vi "SetupCreateObjectFromTree.vi"(8 "error in":errorcluster, 11 "TreeControl in":refnum<vi>) -> (0 "error out":errorcluster, 3 "Setup out":refnum<class "Setup.lvclass">)   [LabVIEW 2013, in "DataCreation.lvlib"]
uses:
  DataCreation.lvlib
  classes/Datastructure/Setup/Setup.lvclass
  classes/Datastructure/Image/img.lvclass
  classes/Datastructure/Device/Device.lvclass
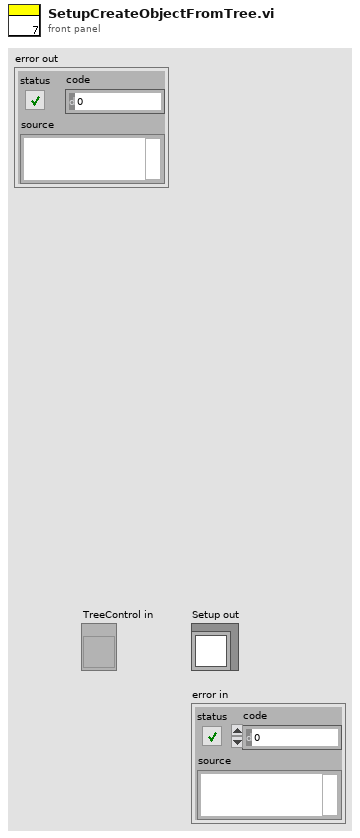
[diagram p1: front panel]
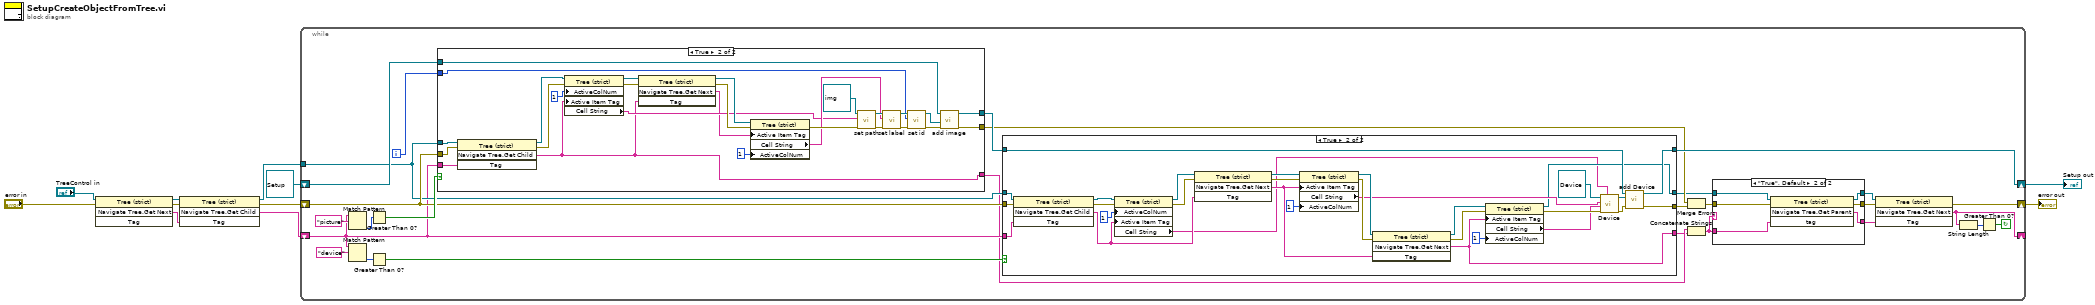
[diagram p0: block diagram]
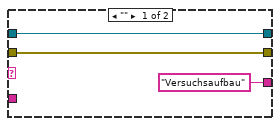
[diagram p2: hidden frame]
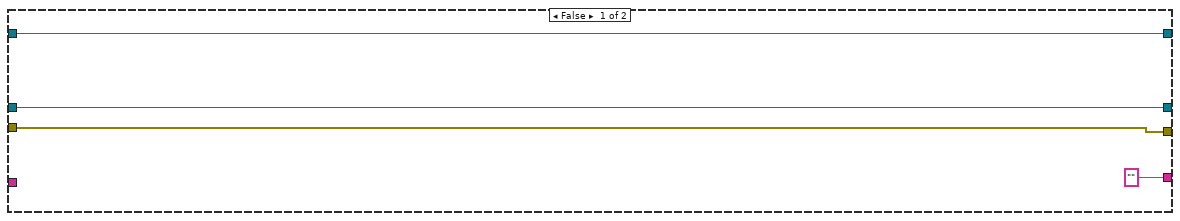
[diagram p3: hidden frame]
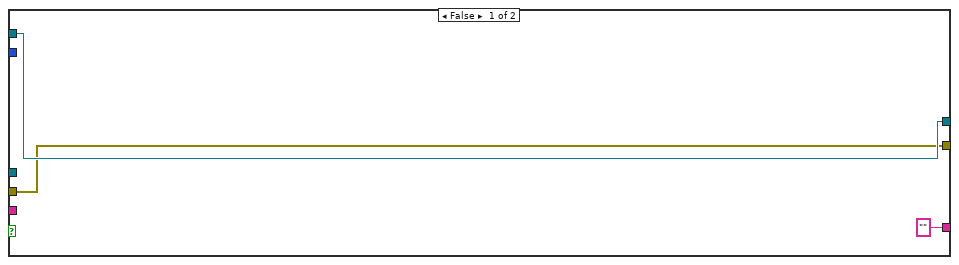
[diagram p4: hidden frame]
diagram:
  n1 = invoke class="Tree (strict)" method="Navigate Tree.Get Next"(reference="TreeControl in", error in="error in") -> (reference out=w6:refnum<vi>, error out=w7:errorcluster, "Navigate Tree:Get Next Item"=w8:string)  [unwired: 2 in, 1 out]
  n2 = invoke class="Tree (strict)" method="Navigate Tree.Get Child"(reference=w6, error in=w7, "Tag"=w8) -> (reference out=w11:refnum<vi>, error out=w9:errorcluster, "Navigate Tree:Get Child"=w10:string)  [unwired: 1 in, 1 out]
  n3 = while {
    shift-right: [w16] -> w1
    shift-left: w9 -> [w32]
    shift-right: [w25] -> w3
    shift-left: refnum<class "Setup.lvclass"> refnum ("Setup Ausgang") -> [w31]
    shift-right: [w14] -> _
    shift-left: w10 -> [w29]
    tunnel: w11 -> [w30]
    i -> [w12]
    stop <- w19 continue-if-true
    n4 = Match Pattern(string=w29, regular expression="picture" ("Regulärer Ausdruck")) -> (offset past match=w37:i32)  [unwired: 1 in, 3 out]
    n5 = Match Pattern(string=w29, regular expression="device" ("Regulärer Ausdruck")) -> (offset past match=w33:i32)  [unwired: 1 in, 3 out]
    n6 = Greater Than 0?(x=w37) -> (x > 0?=w36:bool)
    n7 = Greater Than 0?(x=w33) -> (x > 0?=w35:bool)
    n8 = case shown="True" w36 {
      tunnel: w29 -> [_ w92]
      tunnel: w32 -> [w82 w93]
      tunnel: w30 -> [_ w94]
      tunnel: [w82 w98] -> w24
      tunnel: w31 -> [w83 w97]
      tunnel: [w83 w91] -> w26
      tunnel: ["" ("Navigate Tree:Get Child") w90] -> w28
      tunnel: w12 -> [_ w87]
      frame False {
      }
      frame True {
        n9 = invoke class="Tree (strict)" method="Navigate Tree.Get Child"(reference=w94, error in=w93, "Tag"=w92) -> (reference out=w96:refnum<vi>, error out=w95:errorcluster, "Navigate Tree:Get Child"=w90:string)  [unwired: 1 in, 1 out]
        n10 = property class="Tree (strict)"(reference=w96, error in=w95, "ActiveColNum"=1 ("Active Cell:Active Column Number"), "Active Item Tag"=w90) -> (reference out=w106:refnum<vi>, error out=w107:errorcluster, "Cell String"=w102:string)
        n11 = invoke class="Tree (strict)" method="Navigate Tree.Get Next"(reference=w106, error in=w107, "Tag"=w90) -> (reference out=w105:refnum<vi>, error out=w104:errorcluster, "Navigate Tree:Get Next Item"=w101:string)  [unwired: 1 in, 1 out]
        n12 = property class="Tree (strict)"(reference=w105, error in=w104, "Active Item Tag"=w101, "ActiveColNum"=1 ("Active Cell:Active Column Number")) -> (error out=w111:errorcluster, "Cell String"=w103:string)  [unwired: 1 out]
        n13 = call-dynamic "set path.vi"("error in (no error)"=w111, "path"=w102, "img (Eingang)"=refnum<class "img.lvclass"> refnum ("img.lvclass")) -> ("error out"=w110:errorcluster, "img (Ausgang)"=w108:refnum<class "img.lvclass">)  [unwired: 7 in]
        n14 = call-dynamic "set label.vi"("error in (no error)"=w110, "label"=w103, "img (Eingang)"=w108) -> ("error out"=w88:errorcluster, "img (Ausgang)"=w89:refnum<class "img.lvclass">)  [unwired: 7 in]
        n15 = call-dynamic "set id.vi"("error in (no error)"=w88, "id"=w87, "img in"=w89) -> ("error out"=w86:errorcluster, "img out"=w85:refnum<class "img.lvclass">)  [unwired: 7 in]
        n16 = call-dynamic "add image.vi"("error in (no error)"=w86, "img.lvclass"=w85, "Setup (Eingang)"=w97) -> ("error out"=w98:errorcluster, "Setup (Ausgang)"=w91:refnum<class "Setup.lvclass">)  [unwired: 7 in]
      }
    }
    n17 = case shown="True" w35 {
      tunnel: w32 -> [w49 w74]
      tunnel: w30 -> [w48 w73]
      tunnel: w29 -> [_ w71]
      tunnel: ["" ("Navigate Tree:Get Next Item") w62] -> w27
      tunnel: w26 -> [w50 w56]
      tunnel: [w49 w57] -> w23
      tunnel: [w50 w55] -> w25
      tunnel: [w48 w54] -> w21
      frame False {
      }
      frame True {
        n18 = invoke class="Tree (strict)" method="Navigate Tree.Get Child"(reference=w73, error in=w74, "Tag"=w71) -> (reference out=w72:refnum<vi>, error out=w75:errorcluster, "Navigate Tree:Get Child"=w70:string)  [unwired: 1 in, 1 out]
        n19 = property class="Tree (strict)"(reference=w72, error in=w75, "ActiveColNum"=1 ("Active Cell:Active Column Number"), "Active Item Tag"=w70) -> (reference out=w80:refnum<vi>, error out=w81:errorcluster, "Cell String"=w52:string)
        n20 = invoke class="Tree (strict)" method="Navigate Tree.Get Next"(reference=w80, error in=w81, "Tag"=w70) -> (reference out=w79:refnum<vi>, error out=w78:errorcluster, "Navigate Tree:Get Next Item"=w63:string)  [unwired: 1 in, 1 out]
        n21 = property class="Tree (strict)"(reference=w79, error in=w78, "Active Item Tag"=w63, "ActiveColNum"=1 ("Active Cell:Active Column Number")) -> (reference out=w68:refnum<vi>, error out=w69:errorcluster, "Cell String"=w64:string)
        n22 = invoke class="Tree (strict)" method="Navigate Tree.Get Next"(reference=w68, error in=w69, "Tag"=w63) -> (reference out=w67:refnum<vi>, error out=w66:errorcluster, "Navigate Tree:Get Next Item"=w62:string)  [unwired: 1 in, 1 out]
        n23 = property class="Tree (strict)"(reference=w67, error in=w66, "Active Item Tag"=w62, "ActiveColNum"=1 ("Aktive Zelle:Nummer der aktiven Spalte")) -> (reference out=w54:refnum<vi>, error out=w61:errorcluster, "Cell String"=w53:string)
        n24 = call-dynamic "Device.vi"("last calibration"=w52, "error in (no error)"=w61, "Name"=w53, "serial"=w64, "Device Eingang"=refnum<class "Device.lvclass"> refnum ("Device.lvclass")) -> ("error out"=w58:errorcluster, "Device Ausgang"=w59:refnum<class "Device.lvclass">)  [unwired: 5 in]
        n25 = call-dynamic "add Device.vi"("error in (no error)"=w58, "Device.lvclass"=w59, "Setup Eingang"=w56) -> ("error out"=w57:errorcluster, "Setup Ausgang"=w55:refnum<class "Setup.lvclass">)  [unwired: 7 in]
      }
    }
    n26 = Merge Errors(w24, w23) -> (w22:errorcluster)
    n27 = Concatenate Strings(w28, w27) -> (w13:string)
    n28 = case shown="\"True\", Default" w13 {
      tunnel: w22 -> [w41 w47]
      tunnel: w21 -> [w40 w46]
      tunnel: w13 -> [_ w45]
      tunnel: [w41 w44] -> w18
      tunnel: [w40 w43] -> w17
      tunnel: ["Versuchsaufbau" ("Navigate Tree:Get Parent") w42] -> w15
      frame "" {
      }
      frame "True", Default {
        n29 = invoke class="Tree (strict)" method="Navigate Tree.Get Parent"(reference=w46, error in=w47, "tag"=w45) -> (reference out=w43:refnum<vi>, error out=w44:errorcluster, "Navigate Tree:Get Parent"=w42:string)  [unwired: 1 in, 1 out]
      }
    }
    n30 = invoke class="Tree (strict)" method="Navigate Tree.Get Next"(reference=w17, error in=w18, "Tag"=w15) -> (error out=w16:errorcluster, "Navigate Tree:Get Next Item"=w14:string)  [unwired: 1 in, 2 out]
    n31 = String Length(string=w14) -> (length=w20:i32)
    n32 = Greater Than 0?(x=w20) -> (x > 0?=w19:bool)
  }
  "Setup out" <- w3
  "error out" <- w1
